vi "Evaluate Unsaved Changes.vi"(8 "error in (no error)":errorcluster, 11 "Test Executive Builder Model in":refnum<class "Test Executive Builder Model.lvclass">) -> (0 "error out":errorcluster, 3 "Test Executive Builder Model out":refnum<class "Test Executive Builder Model.lvclass">)   [LabVIEW 2017, in "Test Executive Builder Model.lvclass"]
uses:
  Test Executive Builder Model.lvclass
  <vilib>/gpm_packages/@cs/test-executive/Source/Test Executive/TestExecutive Ref/TestExecutive Ref.lvclass
  <vilib>/gpm_packages/@cs/mva-core/Source/IModel/IModel/IModel.lvclass
  C:/Users/jonmc/Documents/Git/Test Executive Builder/gpm_packages/@cs/mva-core/Source/IModel/IModel/IModel.lvclass
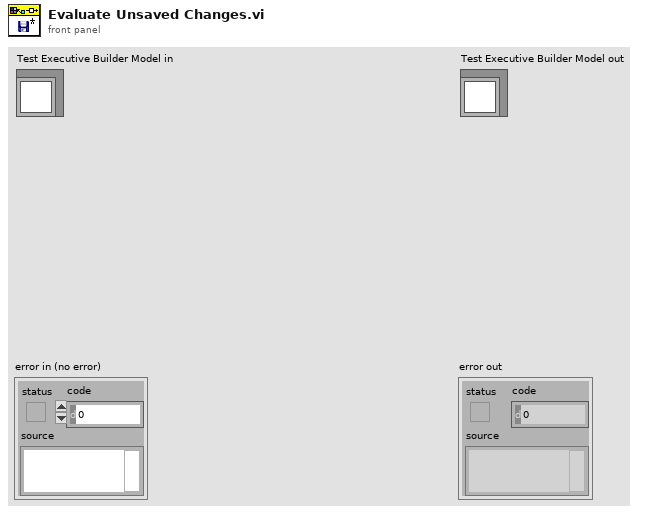
[diagram p1: front panel]
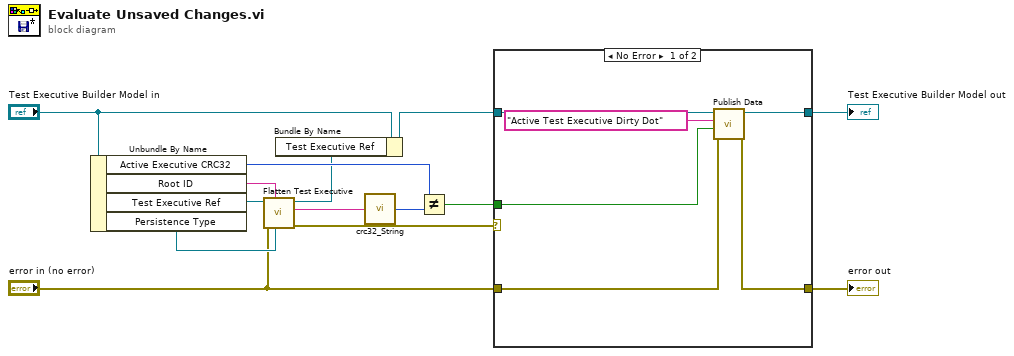
[diagram p0: block diagram]
diagram:
  n1 = Unbundle By Name("Test Executive Builder Model in") -> ("Active Executive CRC32"=w9:u32, "Root ID"=w12:string, "Test Executive Ref"=w13:refnum<data-value>, "Persistence Type"=w11:refnum<class "IPersist.lvclass">)
  n2 = call <vilib>:"Flatten Test Executive.vi"("Persistence in"=w11, "Root ID"=w12, "error in (no error)"="error in (no error)", "Test Executive Ref"=w13) -> ("error out"=w1:errorcluster, "Flattened Test Executive"=w14:string, "Test Executive Ref out"=w7:refnum<data-value>)  [unwired: 5 in]
  n3 = Bundle By Name(cluster="Test Executive Builder Model in", "Test Executive Ref"=w7) -> (w6:refnum<class "Test Executive Builder Model.lvclass">)
  n4 = call "crc32_String.vi"("String in"=w14) -> ("CRC32"=w10:u32)  [unwired: 1 in]
  n5 = Not Equal?(x=w9, y=w10) -> (x != y?=w3:bool)
  n6 = case shown="No Error" w1 {
    tunnel: w6 -> [w20 w22]
    tunnel: [w19 w22] -> w5
    tunnel: [w18 w21] -> w4
    tunnel: w3 -> [w16 _]
    tunnel: "error in (no error)" -> [w15 w21]
    frame No Error {
      n7 = call <vilib>:"Publish Data.vi"("error in (no error)"=w15, "Data to Publish"=w16, "Datum Name"="Active Test Executive Dirty Dot", "IModel in"=w20) -> ("error out"=w18:errorcluster, "IModel out"=w19:refnum<class "Test Executive Builder Model.lvclass">)  [unwired: 6 in]
    }
    frame Error {
    }
  }
  "error out" <- w4
  "Test Executive Builder Model out" <- w5
